vi "3D02_Grab_and_Plot.vi"() -> ()   [LabVIEW 2012]
doc: "The Low-Level Grab Raw Data VI acquires images continuously and displays the images in an image control using low-level acquisition VIs. This VI demonstrates how to acquire raw data from the camera. A grab is appropriate for high-speed applications in which you need to process only one image at a time."
uses:
  <vilib>/userDefined/High Color/IMAQdx.ctl
  <vilib>/vision/driver/IMAQdx.llb/IMAQdx Buffer Number Mode.ctl
  <vilib>/vision/driver/NI_Vision_Acquisition_Software.lvlib
  <resource>/objmgr/imaqdx.rc
  <userlib>/Photonfocus Toolkit/Photonfocus_Toolkit.lvlib
panel:
  in  "NumProfiles":u16=700
  out "Width Profile":u8[][](array[numeric])
  out "Quality Profile":u8[][](array[numeric])
  in  "Tab Control":enum32{"Images", "Maps", "3D View"}(tab)
  out "Image":T1(plugin-control)
  out "Peak":sgl[](graph)
  out "Width":u8[](graph)
  out "Quality":u8[](graph)
  out "Range Map":T1(plugin-control)
  out "Width Map":T1(plugin-control)
  out "Quality Map":T1(plugin-control)
  in  "3D Surface":refnum<k7>(container)
  in  "stop":bool
  out "Peak Profile":sgl[][](array[numeric])
  in  "FrameCombine_Enable":bool
  in  "FrameCombine_NrOfFrames":u32
  in  "PeakDetector_Mode":u32
  in  "Camera Name":T2
  out "Buffer Number":u32
  out "Frame Rate":dbl(knob) scale=0.0..100.0 scale format="%.1f"
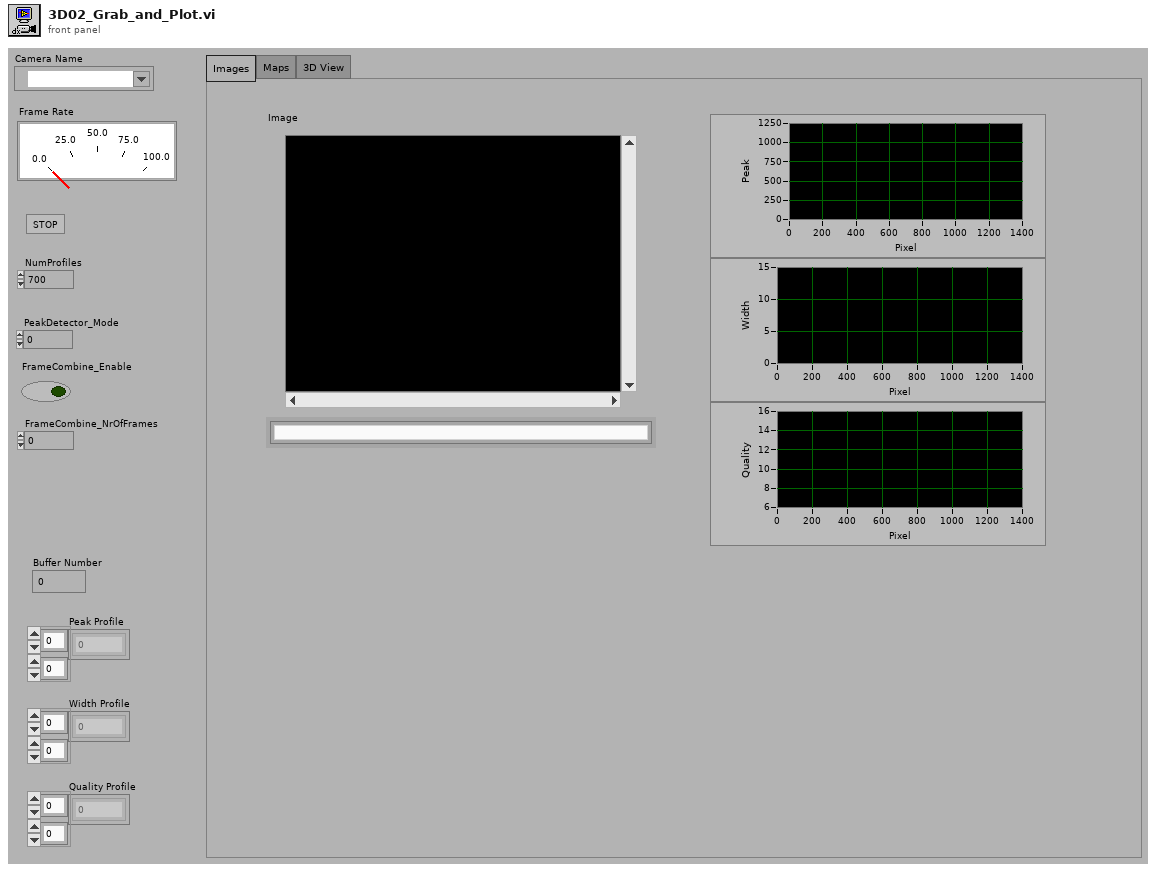
[diagram p1: front panel]
types:
  T1 = typedef "IMAQ Image.ctl" = refnum<image>
  T2 = typedef "IMAQdx.ctl" = refnum<k21>
  T3 = typedef "Image Type" = u32
  T4 = typedef "NI_Vision_Acquisition_Software.lvlib/IMAQdx Buffer Number Mode.ctl" = enum32{"Next", "Last", "Buffer Number"}
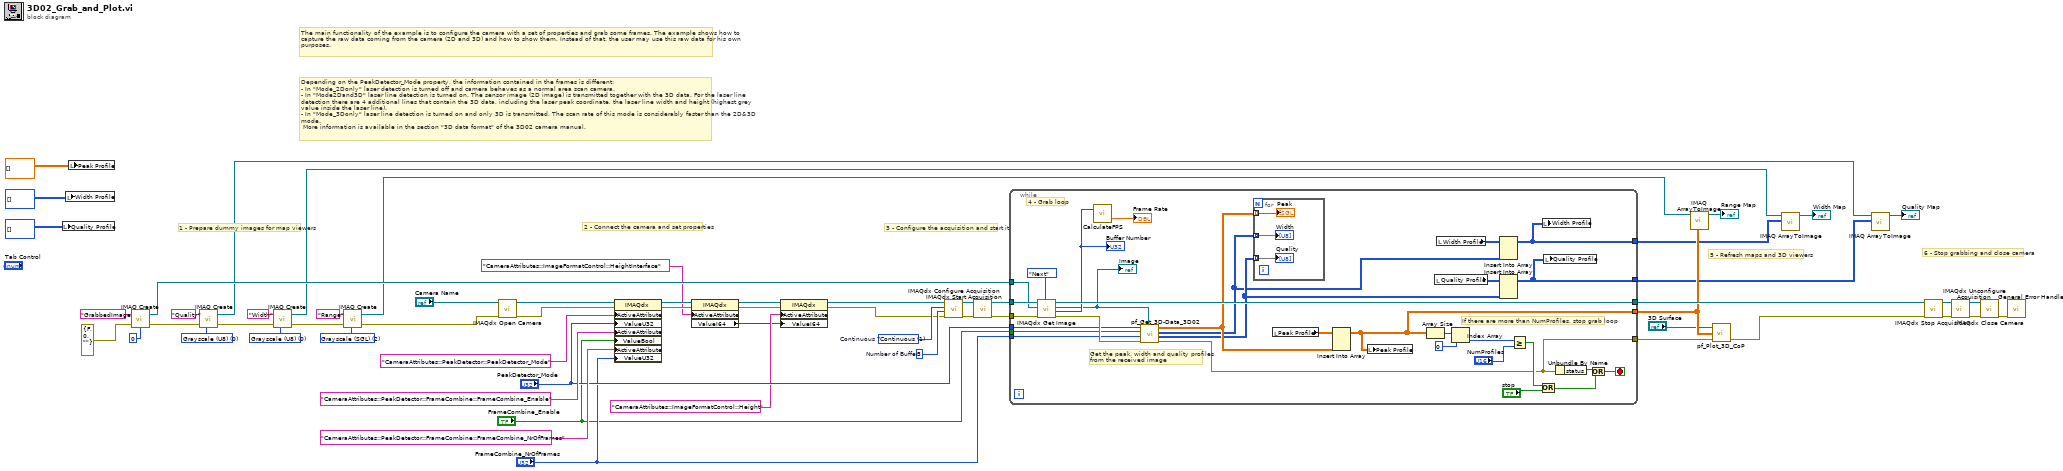
[diagram p0: block diagram]
diagram:
  w14 = T3 2 items=["Grayscale (U8)", "Grayscale (I16)", "Grayscale (SGL)", "Complex (CSG)", "RGB (U32)", "HSL (U32)", "RGB (U64)", "Grayscale (U16)"] ("Image Type")
  w15 = T3 0 items=["Grayscale (U8)", "Grayscale (I16)", "Grayscale (SGL)", "Complex (CSG)", "RGB (U32)", "HSL (U32)", "RGB (U64)", "Grayscale (U16)"] ("Image Type")
  w26 = T3 0 items=["Grayscale (U8)", "Grayscale (I16)", "Grayscale (SGL)", "Complex (CSG)", "RGB (U32)", "HSL (U32)", "RGB (U64)", "Grayscale (U16)"] ("Image Type")
  w55 = u32 3  # Number of Buffer
  w56 = u32 1 items=["One Shot", "Continuous"]  # Continuous ?
  # "Depending on the PeakDetector_Mode property, the information contained in the frames is different:\n- In \"Mode_2Donly\" laser detection is turned off and camera behaves as a normal area scan camera.\n- In \"Mode2Dand3D\" laser line detection is turned on. The sensor image (2D image) is transmitted together with the 3D data. For the laser line detection there are 4 additional lines that contain the 3D data, including the laser peak coordinate, the laser line width and height (highest grey value inside the laser line).\n- In \"Mode_3Donly\" laser line detection is turned on and only 3D is transmitted. The scan rate of this mode is considerably faster than the 2D&3D mode.\n More information is available in the section \"3D data format\" of the 3D02 camera manual."
  # "The main functionality of the example is to configure the camera with a set of properties and grab some frames. The example shows how to capture the raw data coming from the camera (2D and 3D) and how to show them. Instead of that, the user may use this raw data for his own purposes."
  # "6 - Stop grabbing and close camera"
  # "5 - Refresh maps and 3D viewers"
  # "3 - Configure the acquisition and start it"
  # "2 - Connect the camera and set properties"
  # "1 - Prepare dummy images for map viewers"
  n1 = local write "Quality Profile"(u8[][] []) -> ()
  n2 = local write "Width Profile"(u8[][] []) -> ()
  n3 = local write "Peak Profile"(dbl[][] []) -> ()
  n4 = call "IMAQ Create"("Image Name"="GrabbedImage", "Image Type"=0, "error in (no error)"=errorcluster {"status"=FALSE, "code"=0, "source"=""}) -> ("New Image"=w45:T1, "error out"=w25:errorcluster)  [unwired: 1 in, 1 out]
  n5 = call "IMAQ Create"("Image Name"="Quality", "Image Type"=w26, "error in (no error)"=w25) -> ("New Image"=w5:T1, "error out"=w13:errorcluster)  [unwired: 1 in, 1 out]
  n6 = call "IMAQ Create"("Image Name"="Width", "Image Type"=w15, "error in (no error)"=w13) -> ("New Image"=w9:T1, "error out"=w18:errorcluster)  [unwired: 1 in, 1 out]
  n7 = call "IMAQ Create"("Image Name"="Range", "Image Type"=w14, "error in (no error)"=w18) -> ("New Image"=w11:T1, "error out"=w12:errorcluster)  [unwired: 1 in, 1 out]
  n8 = call <vilib>:"IMAQdx Open Camera.vi"("error in"=w12, "Session In"="Camera Name") -> ("error out"=w43:errorcluster, "Session Out"=w44:T2)  [unwired: 1 in, 7 out]
  n9 = property class="IMAQdx"(reference=w44, error in=w43, "ActiveAttribute"="CameraAttributes::PeakDetector::PeakDetector_Mode", "ValueU32"="PeakDetector_Mode", "ActiveAttribute"="CameraAttributes::PeakDetector::FrameCombine::FrameCombine_Enable", "ValueBool"="FrameCombine_Enable", "ActiveAttribute"="CameraAttributes::PeakDetector::FrameCombine::FrameCombine_NrOfFrames", "ValueU32"="FrameCombine_NrOfFrames") -> (reference out=w33:T2, error out=w34:errorcluster)
  n10 = property class="IMAQdx"(reference=w33, error in=w34, "ActiveAttribute"="CameraAttributes::ImageFormatControl::HeightInterface") -> (reference out=w32:T2, error out=w35:errorcluster, "ValueI64"=w29:i64)
  n11 = property class="IMAQdx"(reference=w32, error in=w35, "ActiveAttribute"="CameraAttributes::ImageFormatControl::Height", "ValueI64"=w29) -> (reference out=w31:T2, error out=w36:errorcluster)
  n12 = call <vilib>:"IMAQdx Configure Acquisition.vi"("error in"=w36, "Number of Buffers"=w55, "Continuous?"=w56, "Session In"=w31) -> ("error out"=w58:errorcluster, "Session Out"=w57:T2)  [unwired: 6 out]
  n13 = call <vilib>:"IMAQdx Start Acquisition.vi"("error in"=w58, "Session In"=w57) -> ("error out"=w54:errorcluster, "Session Out"=w53:T2)  [unwired: 8 out]
  n14 = while {
    tunnel: [w88] -> w52
    tunnel: w54 -> [w89]
    tunnel: w53 -> [w90]
    tunnel: [w68] -> w22
    tunnel: w45 -> [w84]
    tunnel: "PeakDetector_Mode" -> [w81]
    tunnel: "FrameCombine_Enable" -> [w80]
    tunnel: "FrameCombine_NrOfFrames" -> [w79]
    tunnel: [w66] -> w20
    tunnel: [w61] -> w8
    tunnel: [w60] -> w6
    stop <- w72 stop-if-true
    # "If there are more than NumProfiles, stop grab loop"
    # "Get the peak, width and quality profiles \nfrom the received image"
    # "4 - Grab loop"
    n15 = call <vilib>:"IMAQdx Get Image.vi"("Buffer Number Mode (Next)"=IMAQdx_Buffer_Number_Mode."Next", "error in"=w89, "Image In"=w84, "Session In"=w90) -> ("error out"=w82:errorcluster, "Buffer Number Out"=w85:u32, "Image Out"=w83:T1, "Session Out"=w88:T2)  [unwired: 4 in]
    "Buffer Number" <- w85
    "Image" <- w83
    n16 = call <userlib>:"CalculateFPS.vi"("buffer number"=w85) -> ("processed FPS"=→"Frame Rate":dbl)  [unwired: 2 out]
    n17 = call <userlib>:"pf_Get_3D-Data_3D02.vi"("Aquired Image"=w83, "error in (no error)"=w82, "FrameCombine_NrOfFrames"=w79, "FrameCombine_Enable"=w80, "PealDetector_Mode"=w81) -> ("error out"=w68:errorcluster, "Quality Profile"=w64:u8[][], "Width Profile"=w62:u8[][], "Peak Profile"=w67:sgl[][])  [unwired: 2 in, 1 out]
    n18 = for {
      tunnel: w67 -> [w93] mode=indexing
      tunnel: w62 -> [w92] mode=indexing
      tunnel: w64 -> [w91] mode=indexing
      "Peak" <- w93
      "Width" <- w92
      "Quality" <- w91
    }
    n19 = local read "Peak Profile"() -> (w78:sgl[][])
    n20 = Insert Into Array "Insert Into Array"(array=w78, new element=w67) -> (w66:sgl[][])  [unwired: 2 in]
    n21 = local write "Peak Profile"(w66) -> ()
    n22 = Array Size(array=w66) -> (size(s)=w77:i32[])
    n23 = local read "Quality Profile"() -> (w65:u8[][])
    n24 = local read "Width Profile"() -> (w63:u8[][])
    n25 = Index Array(array=w77, index=0) -> (element=w75:i32)
    n26 = Insert Into Array(array=w63, new element=w62) -> (w61:u8[][])  [unwired: 2 in]
    n27 = Insert Into Array(array=w65, new element=w64) -> (w60:u8[][])  [unwired: 2 in]
    n28 = Greater Or Equal?(x=w75, y="NumProfiles") -> (x >= y?=w69:bool)
    n29 = Or(x=w69, y="stop") -> (x .or. y?=w71:bool)
    n30 = local write "Width Profile"(w61) -> ()
    n31 = local write "Quality Profile"(w60) -> ()
    n32 = Unbundle By Name(w68) -> ("status"=w73:bool)
    n33 = Or(x=w73, y=w71) -> (x .or. y?=w72:bool)
  }
  n34 = call "IMAQ ArrayToImage"("Image Pixels (Float)"=w20, "Image"=w11) -> ("Image Out"=→"Range Map":T1)  [unwired: 4 in, 5 out]
  n35 = call <userlib>:"pf_Plot_3D_CoP.vi"("error in (no error)"=w22, "Range Map in"=w20, "3D Surface"="3D Surface") -> ("error out"=w21:errorcluster)  [unwired: 2 in]
  n36 = call "IMAQ ArrayToImage"("Image Pixels (U8)"=w8, "Image"=w9) -> ("Image Out"=→"Width Map":T1)  [unwired: 4 in, 5 out]
  n37 = call "IMAQ ArrayToImage"("Image Pixels (U8)"=w6, "Image"=w5) -> ("Image Out"=→"Quality Map":T1)  [unwired: 4 in, 5 out]
  n38 = call <vilib>:"IMAQdx Stop Acquisition.vi"("error in"=w21, "Session In"=w52) -> ("error out"=w51:errorcluster, "Session Out"=w50:T2)  [unwired: 8 out]
  n39 = call <vilib>:"IMAQdx Unconfigure Acquisition.vi"("error in"=w51, "Session In"=w50) -> ("error out"=w48:errorcluster, "Session Out"=w49:T2)  [unwired: 8 out]
  n40 = call <vilib>:"IMAQdx Close Camera.vi"("error in"=w48, "Session In"=w49) -> ("error out"=w59:errorcluster)  [unwired: 9 out]
  n41 = call <vilib>:"General Error Handler.vi"("error in (no error)"=w59) -> ()  [unwired: 1 in, 14 out]
